vi "Remove Object.vi"(8 "error in (no error)":errorcluster, 10 "Object":refnum<class "Object.lvclass">, 11 "Objects in":refnum<class "Objects.lvclass">) -> (0 "error out":errorcluster, 3 "Objects out":refnum<class "Objects.lvclass">)   [LabVIEW 2019, in "HierDAL Library.lvlib" / "Database.lvlib" / "Repositories.lvlib" / "Objects.lvclass"]
uses:
  Objects.lvclass
  Models Library/Object Class/Object.lvclass
  Models Library/Object Class/Object.lvclass/Object.ctl
  Models Library/Object Class/VIs/Get ID.vi
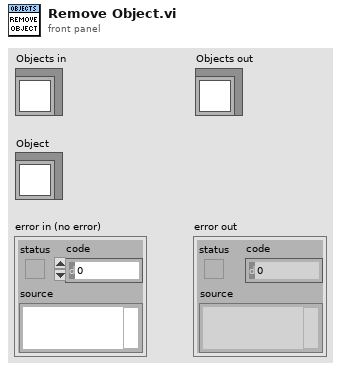
[diagram p1: front panel]
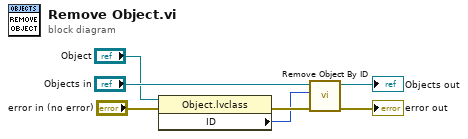
[diagram p0: block diagram]
diagram:
  n1 = property class="Object.lvclass"(reference="Object", error in="error in (no error)") -> (error out=w6:errorcluster, "ID"=w3:i32)  [unwired: 1 out]
  n2 = call "Remove Object By ID.vi"("error in (no error)"=w6, "ID"=w3, "Objects in"="Objects in") -> ("error out"=→"error out":errorcluster, "Objects out"=→"Objects out":refnum<class "Objects.lvclass">)  [unwired: 7 in]
